vi "updateTaskStatus.vi"(8 "error in (no error)":errorcluster, 9 "Status":T1=enum."Added", 10 "Task Name":string, 11 "BuildWorker in":refnum<class "BuildWorker.lvclass">) -> (0 "error out":errorcluster, 3 "BuildWorker out":refnum<class "BuildWorker.lvclass">)   [LabVIEW 2017, in "BuildWorker.lvlib" / "BuildWorker.lvclass"]
uses:
  BuildWorker.lvclass
  Classes/Task/Task.lvclass
  Classes/Task/Status.ctl
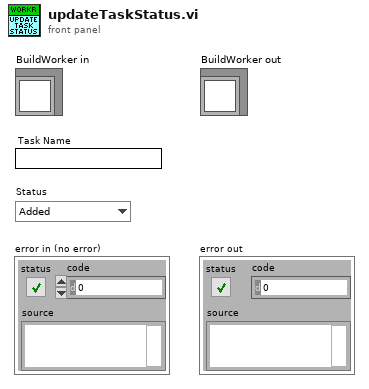
[diagram p1: front panel]
types:
  T1 = typedef "Task Interface.lvlib/Task.lvclass/Status.ctl" = enum16{"Created", "Added", "Pending", "Queued", "Processing", "Cleaning", "Building", "Finished", "Failed", "Removed", "Not found"}
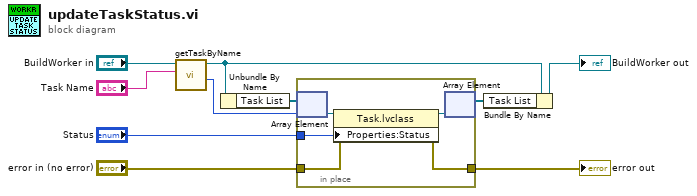
[diagram p0: block diagram]
diagram:
  n1 = call "getTaskByName.vi"("Task Name"="Task Name", "BuildWorker in"="BuildWorker in") -> ("index of element"=w3:i32, "BuildWorker out"=w1:refnum<class "BuildWorker.lvclass">)  [unwired: 7 in, 1 out]
  n2 = Unbundle By Name(w1) -> ("Task List"=w2:refnum<class "Task.lvclass">[])
  n3 = in-place {
    in-place-border: "error in (no error)" -> [w12]
    in-place-border: [w13] -> w10
    in-place-border: "Status" -> [w11]
    n4 = in-place-array #1(w2, w3) -> (w15:refnum<class "Task.lvclass">)
    n5 = property class="Task.lvclass"(reference=w15, error in=w12, "Properties:Status"=w11) -> (reference out=w14:refnum<class "Task.lvclass">, error out=w13:errorcluster)
    n6 = in-place-array #1(w14) -> (w4:refnum<class "Task.lvclass">[])  [unwired: 1 out]
  }
  "error out" <- w10
  n7 = Bundle By Name(cluster=w1, "Task List"=w4) -> (→"BuildWorker out":refnum<class "BuildWorker.lvclass">)
